vi "Proyecto_1er_Parcial_Autotronica_Nicolas_Garces_David_Mera_Anthony_Rogel_David_Mera.vi"() -> ()   [LabVIEW 2026]
uses:
  <vilib>/MakerHub/LINX/LMH-LINX.lvlib
  <vilib>/MakerHub/LINX/Public/Peripherals/Analog/Analog Read 1 Chan.vi
  <vilib>/MakerHub/LINX/Public/Peripherals/Digital/Digital Read 1 Chan.vi
  <vilib>/express/express signal manip/GetorSetDDTAttributes/Set DDT Attributes/Set DDT Properties.xnode
  <vilib>/express/express shared/transition.llb/Dynamic To Waveform Array.vi
  <vilib>/express/express signal manip/GetorSetDDTAttributes/Set DDT Attributes/SetT0.vi
  <vilib>/express/express shared/transition.llb/Waveform Array To Dynamic.vi
  <vilib>/MakerHub/LINX/Public/Utilities/Open Serial.vi
  <vilib>/express/express arith-compare/Formula/XNode/ExpressFormulaBlockNode.xnode
  <vilib>/MakerHub/LINX/Private/Type Defs/Platform.ctl
  <vilib>/MakerHub/LINX/Private/Type Defs/Interface.ctl
  <vilib>/MakerHub/LINX/Private/Device/Type Defs/TCP Config.ctl
  <vilib>/MakerHub/LINX/Private/Device/Device.lvlib
  <vilib>/MakerHub/LINX/Private/Device/Type Defs/Channels.ctl
  <vilib>/MakerHub/LINX/Private/Device/Type Defs/LINX Device Config.ctl
  <vilib>/MakerHub/LINX/Private/Type Defs/LINX Ref.ctl
panel:
  out "BAR 3":dbl
  out "Puerta Piloto":bool
  in  "Serial Port":refnum<visa-resource-name>="N/A"
  in  "stop 2":bool
  out "BAR 2":dbl
  out "BAR":dbl
  out "Millas/h":dbl
  out "BAR 1":dbl
  out "Presion Minima Neumatico Derecho Trasero":bool
  out "Puerta Pasajeros trasero":bool
  out "Puerta Copiloto":bool
  out "Presion Minima Neumatico Izquierdo Trasero":bool
  out "Presion Minima Neumatico Derecho Delantero":bool
  out "Velocidad Maxima":bool
  out "Presion Minima Neumatico Izquierdo Delanterio":bool
  out "PRESION DE NEUMATICO DERECHO TRASERO":dbl(knob) scale=0.0..40.0
  out "PRESION DE NEUMATICO DERECHO DELANTERO":dbl(knob) scale=0.0..40.0
  out "PRESION DE NEUMATICO IZQUIERDO DELANTERO":dbl(knob) scale=0.0..40.0
  out "PRESION DE NEUMATICO IZQUIERDO TRASERO":dbl(knob) scale=0.0..40.0
  out "VELOCIDAD DEL VEHICULO EN KM/H - Millas/h":dbl(knob) scale=0.0..200.0
  # "PSI1"
  # "KM/h"
  # "PSI"
  # "Km"
  # "PSI"
  # "PSI"
  # "PSI"
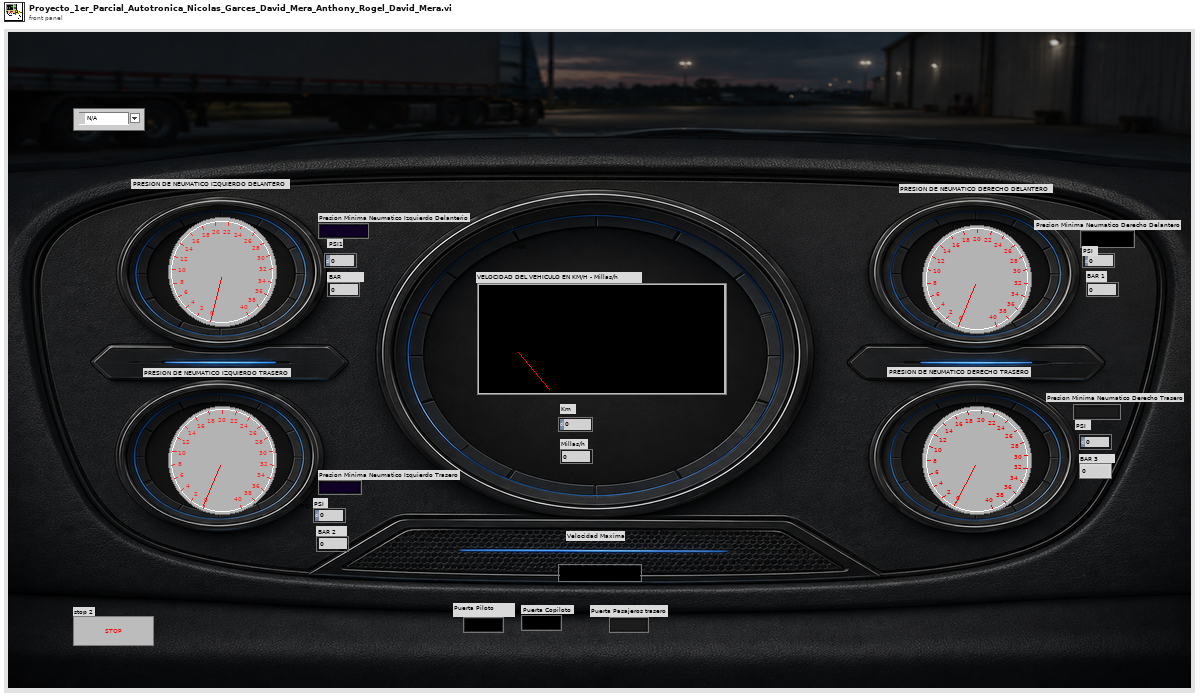
[diagram p1: front panel]
types:
  T1 = typedef "LMH-LINX.lvlib/LINX Ref.ctl" = cluster{"IO":T2, "Interface":T3, "LINX Device Config":T4}
  T2 = typedef "LMH-LINX.lvlib/Platform.ctl" = enum16{"Remote", "Local"}
  T3 = typedef "LMH-LINX.lvlib/Interface.ctl" = enum16{"Serial", "TCP"}
  T4 = typedef "LMH-LINX.lvlib/Device.lvlib/LINX Device Config.ctl" = cluster{"Interface":T3, "COM Port":refnum<visa-resource-name>, "TCP Configuration":T5, "Device Family":u8, "Device ID":u8, "Device Name":string, "TCP Ref":refnum<k5>, "Channels":T6}
  T5 = typedef "LMH-LINX.lvlib/Device.lvlib/TCP Config.ctl" = cluster{"IP Address":string, "Port":u16}
  T6 = typedef "LMH-LINX.lvlib/Channels.ctl" = cluster{"DI":u8[], "DO":u8[], "AI":u8[], "AO":u8[], "PWM":u8[], "QE":u8[], "UART":u8[], "I2C 2":u8[], "SPI":u8[], "CAN":u8[], "Servo":u8[], "AI Ref (V)":dbl, "AI Resolution (Bits)":u8, "AO Ref (V)":dbl, "AO Resolution (Bits)":u8}
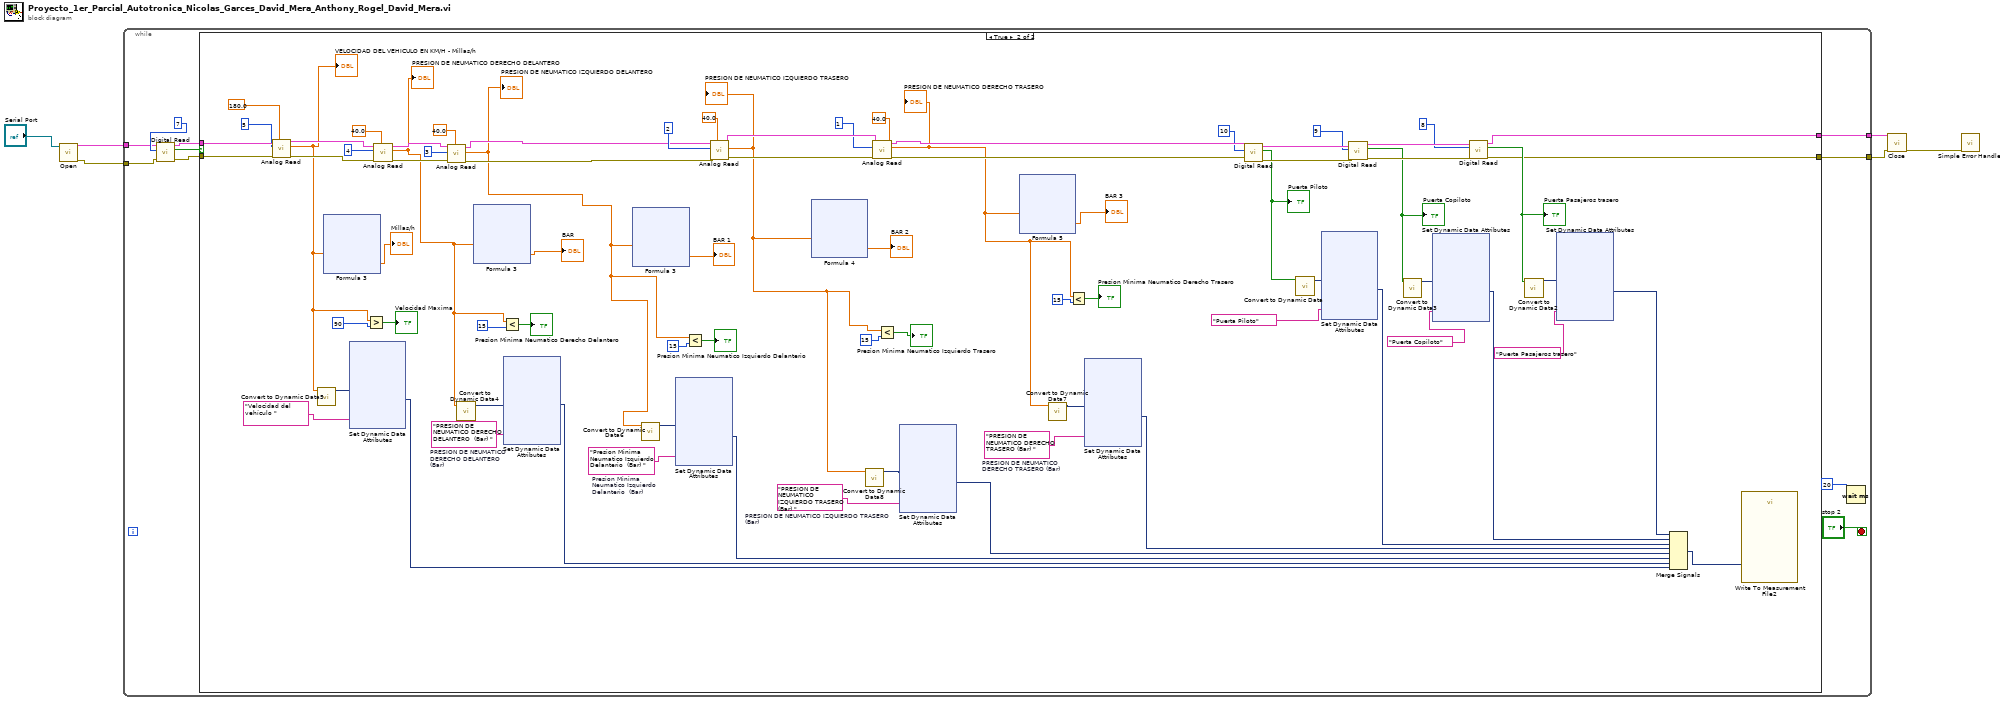
[diagram p0: block diagram]
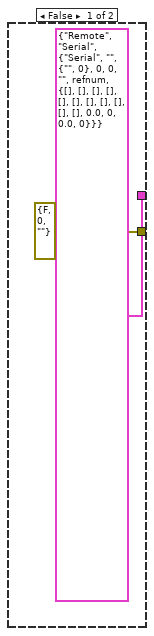
[diagram p2: hidden frame]
diagram:
  n1 = call-poly <vilib>:"Open.vi"("Serial Port"="Serial Port") -> ("Error Out"=w5:errorcluster, "LINX Resource"=w1:T1)  [unwired: 8 in, 1 out]
  n2 = while {
    tunnel: w5 -> [w15]
    tunnel: [w10] -> w3
    tunnel: [w9] -> w2
    tunnel: w1 -> [w8]
    stop <- "stop 2" stop-if-true
    n3 = call-poly <vilib>:"Digital Read.vi"("Error In"=w15, "DI Channel"=7, "LINX Resource"=w8) -> ("Error Out"=w13:errorcluster, "DI Value"=w7:bool, "LINX Resource"=w14:T1)  [unwired: 6 in]
    n4 = case shown="True" w7 {
      tunnel: w14 -> [_ w86]
      tunnel: w13 -> [_ w84]
      tunnel: [T1 {"IO"=enum."Remote", "Interface"=enum."Serial", "LINX Device Config"={"Interface"=enum."Serial", "COM Port"="", "TCP Configuration"={"IP Address"="", "Port"=0}, "Device Family"=0, "Device ID"=0, "Device Name"="", "TCP Ref"=refnum, "Channels"={"DI"=[], "DO"=[], "AI"=[], "AO"=[], "PWM"=[], "QE"=[], "UART"=[], "I2C 2"=[], "SPI"=[], "CAN"=[], "Servo"=[], "AI Ref (V)"=0.0, "AI Resolution (Bits)"=0, "AO Ref (V)"=0.0, "AO Resolution (Bits)"=0}}} ("LINX Resource") w31] -> w10
      tunnel: [errorcluster {"status"=FALSE, "code"=0, "source"=""} ("Error Out") w30] -> w9
      frame False {
      }
      frame True {
        w38 = "PRESION DE NEUMATICO DERECHO TRASERO (Bar) "  # PRESION DE NEUMATICO DERECHO TRASERO (Bar)
        w39 = "PRESION DE NEUMATICO IZQUIERDO TRASERO  (Bar) "  # PRESION DE NEUMATICO IZQUIERDO TRASERO  (Bar)
        w47 = "Presion Minima Neumatico Izquierdo Delanterio  (Bar) "  # Presion Minima Neumatico Izquierdo Delanterio  (Bar)
        w53 = "PRESION DE NEUMATICO DERECHO DELANTERO  (Bar) "  # PRESION DE NEUMATICO DERECHO DELANTERO  (Bar)
        n5 = call-poly <vilib>:"Analog Read.vi"("Analog Ref Override (V)"=180.0, "Error In"=w84, "Analog Channel"=5, "LINX Resource"=w86) -> ("Error Out"=w83:errorcluster, "Voltage"=w58:dbl, "LINX Resource"=w82:T1)  [unwired: 4 in, 1 out]
        "VELOCIDAD DEL VEHICULO EN KM/H - Millas/h" <- w58
        n6 = call "Convert to Dynamic Data5"("Double"=w58) -> ("Dynamic Data Type"=w60:dynamicdata)  [unwired: 3 in]
        n7 = xnode "Formula 3"("X1"=w58) -> ("Result"=→"Millas/h":dbl)  [unwired: 1 in, 1 out]
        n8 = xnode "Set Dynamic Data Attributes"("Signals In"=w60, "Signal Name"="Velocidad del vehículo ") -> ("Signals Out"=w36:dynamicdata)  [unwired: 2 in, 1 out]
        n9 = Greater?(x=w58, y=90) -> (0:→"Velocidad Maxima":bool)
        n10 = call-poly <vilib>:"Analog Read.vi"("Analog Ref Override (V)"=40.0, "Error In"=w83, "Analog Channel"=4, "LINX Resource"=w82) -> ("Error Out"=w80:errorcluster, "Voltage"=w55:dbl, "LINX Resource"=w81:T1)  [unwired: 4 in, 1 out]
        "PRESION DE NEUMATICO DERECHO DELANTERO" <- w55
        n11 = call-poly <vilib>:"Analog Read.vi"("Analog Ref Override (V)"=40.0, "Error In"=w80, "Analog Channel"=3, "LINX Resource"=w81) -> ("Error Out"=w79:errorcluster, "Voltage"=w46:dbl, "LINX Resource"=w78:T1)  [unwired: 4 in, 1 out]
        "PRESION DE NEUMATICO IZQUIERDO DELANTERO" <- w46
        n12 = call "Convert to Dynamic Data4"("Double"=w55) -> ("Dynamic Data Type"=w56:dynamicdata)  [unwired: 3 in]
        n13 = xnode "Formula 3"("X1"=w55) -> ("Result"=→"BAR":dbl)  [unwired: 1 in, 1 out]
        n14 = Less?(x=w55, y=15) -> (x < y?=→"Presion Minima Neumatico Derecho Delantero":bool)
        n15 = xnode "Set Dynamic Data Attributes"("Signals In"=w56, "Signal Name"=w53) -> ("Signals Out"=w35:dynamicdata)  [unwired: 2 in, 1 out]
        n16 = xnode "Formula 3"("X1"=w46) -> ("Result"=→"BAR 1":dbl)  [unwired: 1 in, 1 out]
        n17 = call "Convert to Dynamic Data6"("Double"=w46) -> ("Dynamic Data Type"=w48:dynamicdata)  [unwired: 3 in]
        n18 = xnode "Set Dynamic Data Attributes"("Signals In"=w48, "Signal Name"=w47) -> ("Signals Out"=w34:dynamicdata)  [unwired: 2 in, 1 out]
        n19 = Less?(x=w46, y=15) -> (x < y?=→"Presion Minima Neumatico Izquierdo Delanterio":bool)
        n20 = call-poly <vilib>:"Analog Read.vi"("Analog Ref Override (V)"=40.0, "Error In"=w79, "Analog Channel"=2, "LINX Resource"=w78) -> ("Error Out"=w96:errorcluster, "Voltage"=w19:dbl, "LINX Resource"=w97:T1)  [unwired: 4 in, 1 out]
        "PRESION DE NEUMATICO IZQUIERDO TRASERO" <- w19
        n21 = xnode "Formula 4"("X1"=w19) -> ("Result"=→"BAR 2":dbl)  [unwired: 1 in, 1 out]
        n22 = call "Convert to Dynamic Data8"("Double"=w19) -> ("Dynamic Data Type"=w20:dynamicdata)  [unwired: 3 in]
        n23 = call-poly <vilib>:"Analog Read.vi"("Analog Ref Override (V)"=40.0, "Error In"=w96, "Analog Channel"=1, "LINX Resource"=w97) -> ("Error Out"=w76:errorcluster, "Voltage"=w22:dbl, "LINX Resource"=w77:T1)  [unwired: 4 in, 1 out]
        "PRESION DE NEUMATICO DERECHO TRASERO" <- w22
        n24 = Less?(x=w19, y=15) -> (x < y?=→"Presion Minima Neumatico Izquierdo Trasero":bool)
        n25 = xnode "Set Dynamic Data Attributes"("Signals In"=w20, "Signal Name"=w39) -> ("Signals Out"=w33:dynamicdata)  [unwired: 2 in, 1 out]
        n26 = xnode "Formula 5"("X1"=w22) -> ("Result"=→"BAR 3":dbl)  [unwired: 1 in, 1 out]
        n27 = call "Convert to Dynamic Data7"("Double"=w22) -> ("Dynamic Data Type"=w21:dynamicdata)  [unwired: 3 in]
        n28 = Less?(x=w22, y=15) -> (x < y?=→"Presion Minima Neumatico Derecho Trasero":bool)
        n29 = xnode "Set Dynamic Data Attributes"("Signals In"=w21, "Signal Name"=w38) -> ("Signals Out"=w32:dynamicdata)  [unwired: 2 in, 1 out]
        n30 = call-poly <vilib>:"Digital Read.vi"("Error In"=w76, "DI Channel"=10, "LINX Resource"=w77) -> ("Error Out"=w72:errorcluster, "DI Value"=w70:bool, "LINX Resource"=w74:T1)  [unwired: 6 in]
        "Puerta Piloto" <- w70
        n31 = call "Convert to Dynamic Data"("Boolean"=w70) -> ("Dynamic Data Type"=w87:dynamicdata)  [unwired: 3 in]
        n32 = xnode "Set Dynamic Data Attributes"("Signals In"=w87, "Signal Name"="Puerta Piloto") -> ("Signals Out"=w29:dynamicdata)  [unwired: 2 in, 1 out]
        n33 = call-poly <vilib>:"Digital Read.vi"("Error In"=w72, "DI Channel"=9, "LINX Resource"=w74) -> ("Error Out"=w71:errorcluster, "DI Value"=w68:bool, "LINX Resource"=w73:T1)  [unwired: 6 in]
        "Puerta Copiloto" <- w68
        n34 = call "Convert to Dynamic Data3"("Boolean"=w68) -> ("Dynamic Data Type"=w69:dynamicdata)  [unwired: 3 in]
        n35 = xnode "Set Dynamic Data Attributes"("Signals In"=w69, "Signal Name"="Puerta Copiloto") -> ("Signals Out"=w28:dynamicdata)  [unwired: 2 in, 1 out]
        n36 = call-poly <vilib>:"Digital Read.vi"("Error In"=w71, "DI Channel"=8, "LINX Resource"=w73) -> ("Error Out"=w30:errorcluster, "DI Value"=w66:bool, "LINX Resource"=w31:T1)  [unwired: 6 in]
        "Puerta Pasajeros trasero" <- w66
        n37 = call "Convert to Dynamic Data2"("Boolean"=w66) -> ("Dynamic Data Type"=w67:dynamicdata)  [unwired: 3 in]
        n38 = xnode "Set Dynamic Data Attributes"("Signals In"=w67, "Signal Name"="Puerta Pasajeros trasero") -> ("Signals Out"=w27:dynamicdata)  [unwired: 2 in, 1 out]
        n39 = Merge Signals(w27, w28, w29, w32, w33, w34, w35, w36) -> (w37:dynamicdata)
        n40 = call "Write To Measurement File2"("Signals"=w37) -> ()  [unwired: 16 in, 3 out]
      }
    }
    n41 = Wait (ms)(milliseconds to wait=20) -> ()  [unwired: 1 out]
  }
  n42 = call <vilib>:"Close.vi"("Error In"=w2, "LINX Resource"=w3) -> ("Error Out"=w4:errorcluster)  [unwired: 9 in]
  n43 = call <vilib>:"Simple Error Handler.vi"("error in (no error)"=w4) -> ()  [unwired: 4 in, 5 out]
